vi "Set Light Tree.vi"(10 "Select Light":T1(ring)) -> ()   [LabVIEW 2010]
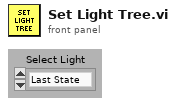
[diagram p1: front panel]
types:
  T1 = enum16{"Last State", "Green Light", "Yellow Light", "Red Light", "None"}
  T2 = enum16{"--Disconnect All--", "Connect PulseGen to CH1", "Connect PulseGen to CH2", "Connect PulseGen to CH3", "Connect PulseGen to CH4", "Connect PulseGen to CH5", "Connect PulseGen to CH6", "Connect PulseGen to CH7", "Connect PulseGen to CH8", "Connect PulseGen to CH9", "Connect PulseGen to CH10", "Connect PulseGen to CH11", "Connect PulseGen to CH12", "Connect PulseGen to CH13", "Connect PulseGen to CH14", "Connect PulseGen to CH15", "Connect PulseGen to CH16", "Connect PulseGen to CH17", "Connect PulseGen to CH18", "Connect PulseGen to CH19", "Connect PulseGen to CH20", "Connect PulseGen to CH21", "Connect PulseGen to CH22", "Connect PulseGen to CH23", "Connect PulseGen to CH24", "Connect PulseGen to CH25", "Set MAG_SW", "Set Dynamic Load", "Set Expansion Trigger", "Trigger Positive Pulse", "Trigger Negative Pulse", "Set MSP Magic Pin", "Set BAT_EN", "Connect MSP_ACLK to CTR", "Connect MSP_MCLK to CTR", "Connect MSP_DIG_TST_OUT to CTR", "Connect STIM_SCK to CTR", "Connect STIM_CLK to CTR", "Connect SMU2 to Magnet", "Magnet Enable", "Cap Short", "Connect Positive Pulse to Pulse Bus", "Connect Negative Pulse to Pulse Bus", "Connect JTAG", "Connect JTAG DVDD Power", "RF Attach", "Connect SMU3 to VBAT", "Connect SMU3 Soft Start", "Connect ARB to Charge Coil", "Connect ARB to Matrix", "Connect CTR to Matrix", "DMM_I Short", "DMM_I 1000 Ohm", "DMM_I 100 Ohm", "DMM_I 10 Ohm", "Connect CH25 to DUT GND", "Enclosure Lights", "Heat Fan Zone 1", "Heat Fan Zone 2", "Temp Zone 1", "Temp Zone 2", "Temp Zone 3", "Guard Door Locks", "Air Heat Zone 3", "Zone 3 Vent", "Zone 3 Loader", "Zone 3 Upper Bed", "Zone 3 Lower Bed", "Zone 3 Standby Temp", "Yellow Light", "Red Light", "Green Light", "Reset Common Test Lines"}
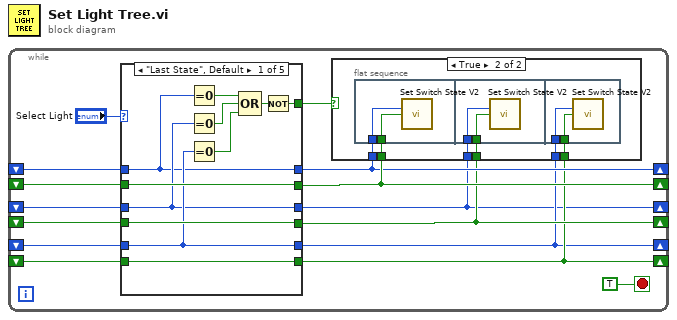
[diagram p0: block diagram]
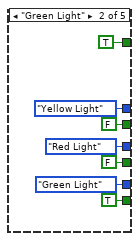
[diagram p3: hidden frame]
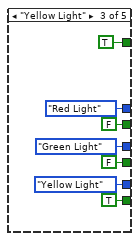
[diagram p4: hidden frame]
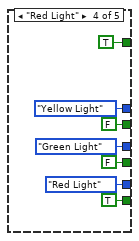
[diagram p5: hidden frame]
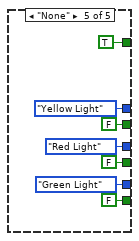
[diagram p6: hidden frame]
diagram:
  n1 = while {
    shift-right: [w5] -> _
    shift-left: _ -> [w14]
    shift-right: [w6] -> _
    shift-left: _ -> [w13]
    shift-right: [w1] -> _
    shift-left: _ -> [w12]
    shift-right: [w4] -> _
    shift-left: _ -> [w11]
    shift-right: [w2] -> _
    shift-left: _ -> [w10]
    shift-right: [w3] -> _
    shift-left: _ -> [w9]
    stop <- TRUE stop-if-true
    n2 = case shown="\"Last State\", Default" "Select Light" {
      tunnel: [w30 T2."Green Light" ("Action") T2."Yellow Light" ("Action") T2."Red Light" ("Action") T2."Green Light" ("Action")] -> w2
      tunnel: [w36 TRUE TRUE TRUE FALSE] -> w3
      tunnel: [w28 T2."Yellow Light" ("Action") T2."Red Light" ("Action") T2."Yellow Light" ("Action") T2."Yellow Light" ("Action")] -> w5
      tunnel: [w38 FALSE FALSE FALSE FALSE] -> w6
      tunnel: [w29 T2."Red Light" ("Action") T2."Green Light" ("Action") T2."Green Light" ("Action") T2."Red Light" ("Action")] -> w1
      tunnel: [w37 FALSE FALSE FALSE FALSE] -> w4
      tunnel: w14 -> [w28 _ _ _ _]
      tunnel: w13 -> [w38 _ _ _ _]
      tunnel: w12 -> [w29 _ _ _ _]
      tunnel: w11 -> [w37 _ _ _ _]
      tunnel: w10 -> [w30 _ _ _ _]
      tunnel: w9 -> [w36 _ _ _ _]
      tunnel: [w31 TRUE TRUE TRUE TRUE] -> w7
      frame "Last State", Default {
        n3 = Equal To 0?(x=w28) -> (x = 0?=w34:bool)
        n4 = Equal To 0?(x=w29) -> (x = 0?=w33:bool)
        n5 = Equal To 0?(x=w30) -> (x = 0?=w32:bool)
        n6 = Compound Arithmetic op=OR(w34, w33, w32) -> (w35:bool)
        n7 = Not(x=w35) -> (.not. x?=w31:bool)
      }
      frame "Green Light" {
      }
      frame "Yellow Light" {
      }
      frame "Red Light" {
      }
      frame "None" {
      }
    }
    n8 = case shown="True" w7 {
      tunnel: w6 -> [_ w21]
      tunnel: w5 -> [_ w20]
      tunnel: w4 -> [_ w19]
      tunnel: w1 -> [_ w18]
      tunnel: w3 -> [_ w17]
      tunnel: w2 -> [_ w16]
      frame False {
      }
      frame True {
        n9 = flat-sequence {
          tunnel: w20 -> [w23]
          tunnel: w21 -> [w22]
          tunnel: w18 -> [w25]
          tunnel: w19 -> [w24]
          tunnel: w16 -> [w27]
          tunnel: w17 -> [w26]
          frame #0 {
            n10 = call "Set Switch State V2.vi"("Action"=w23, "State"=w22) -> ()  [unwired: 13 in, 1 out]
          }
          frame #1 {
            n11 = call "Set Switch State V2.vi"("Action"=w25, "State"=w24) -> ()  [unwired: 13 in, 1 out]
          }
          frame #2 {
            n12 = call "Set Switch State V2.vi"("Action"=w27, "State"=w26) -> ()  [unwired: 13 in, 1 out]
          }
        }
      }
    }
  }
